vi "Write Cmd Parameters.vi"(8 "error in (no error)":errorcluster, 10 "Cmd Parameters":string, 11 "HIJ Vision Launcher in":refnum<class "HIJ Vision Launcher.lvclass">) -> (0 "error out":errorcluster, 3 "HIJ Vision Launcher out":refnum<class "HIJ Vision Launcher.lvclass">)   [LabVIEW 2014, in "HIJ Vision Launcher.lvlib" / "HIJ Vision Launcher.lvclass"]
uses:
  HIJ Vision Launcher.lvclass
  HIJ Vision Launcher.lvclass/HIJ Vision Launcher.ctl
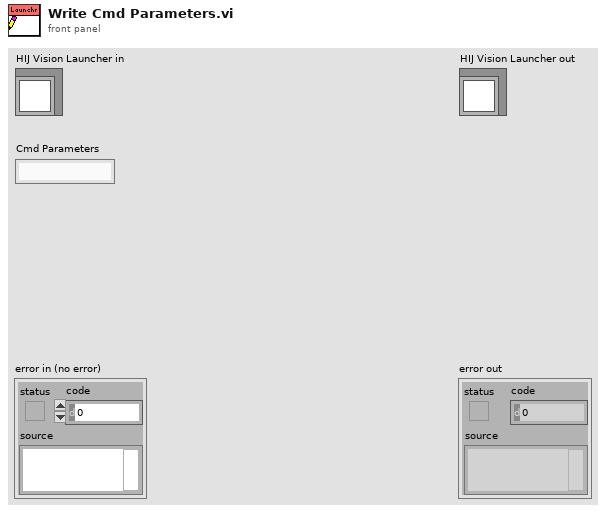
[diagram p1: front panel]
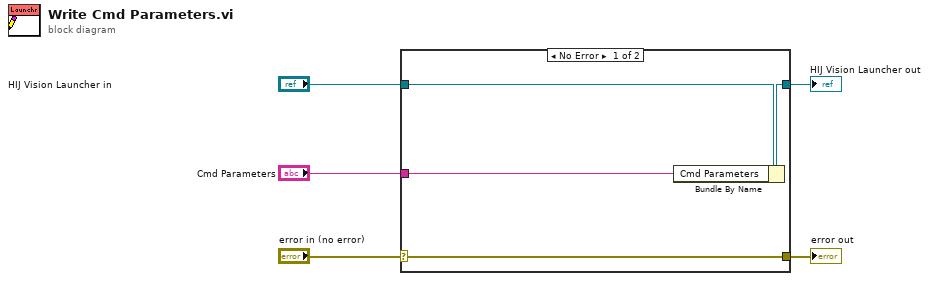
[diagram p0: block diagram]
diagram:
  n1 = case shown="No Error" "error in (no error)" {
    selector: "error in (no error)" -> [w9 w10]
    tunnel: [w9 w10] -> w4
    tunnel: [w7 w11] -> w2
    tunnel: "HIJ Vision Launcher in" -> [w8 w11]
    tunnel: "Cmd Parameters" -> [w6 _]
    frame No Error {
      n2 = Bundle By Name(cluster=w8, "Cmd Parameters"=w6) -> (w7:refnum<class "HIJ Vision Launcher.lvclass">)
    }
    frame Error {
    }
  }
  "error out" <- w4
  "HIJ Vision Launcher out" <- w2
